vi "Script Constant VI.vi"(7 "Custom Argument Window":refnum<vi>, 8 "error in":errorcluster, 11 "VI Reference":refnum<vi>) -> (0 "error out":errorcluster, 3 "VI reference":refnum<vi>)   [LabVIEW 2019, in "Panther Dashboard.lvlib"]
uses:
  Panther Dashboard.lvlib
  <vilib>/Utility/traverseref.llb/TRef TravTarget.ctl
  <vilib>/Utility/miscctls.llb/LVPositionTypeDef.ctl
  <vilib>/Utility/traverseref.llb/VI Scripting - Traverse.lvlib
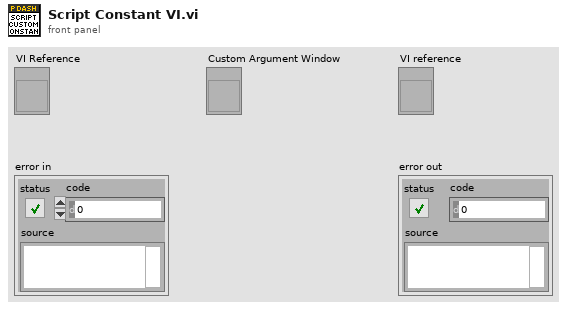
[diagram p1: front panel]
types:
  T1 = typedef "TRef TravTarget.ctl" = enum16{"FP", "BD", "Other"}
  T2 = typedef "LVPositionTypeDef.ctl" = cluster{"Left":i32, "Top":i32}
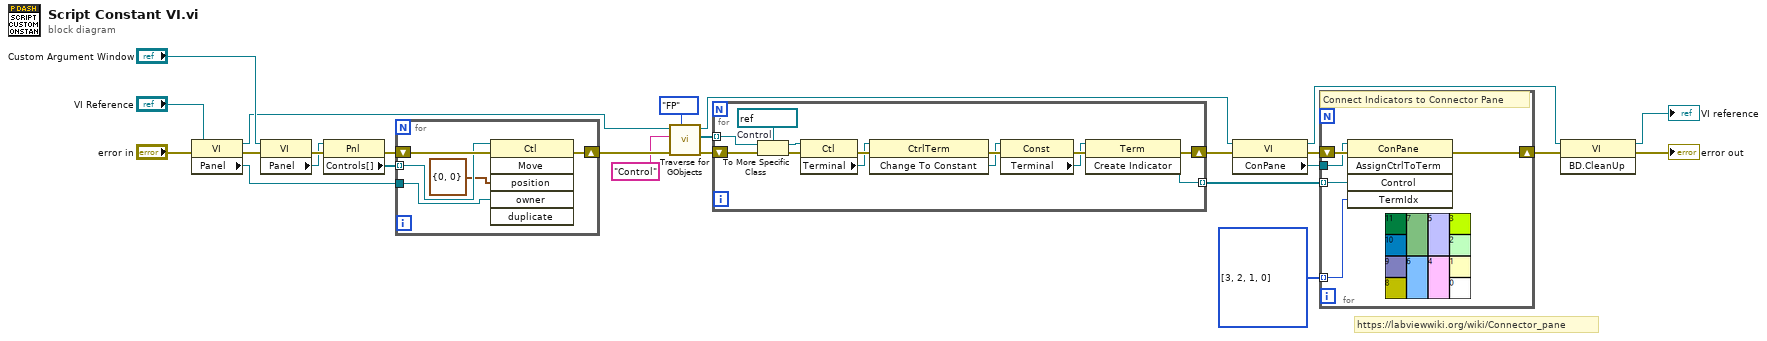
[diagram p0: block diagram]
diagram:
  # "https://labviewwiki.org/wiki/Connector_pane"
  n1 = property class="VI"(reference="VI Reference", error in="error in") -> (reference out=w9:refnum<vi>, error out=w22:errorcluster, "Panel"=w12:refnum<vi>)
  n2 = property class="VI"(reference="Custom Argument Window", error in=w22) -> (error out=w24:errorcluster, "Panel"=w14:refnum<vi>)  [unwired: 1 out]
  n3 = property class="Pnl"(reference=w14, error in=w24) -> (error out=w23:errorcluster, "Controls[]"=w13:refnum<vi>[])  [unwired: 1 out]
  n4 = for {
    tunnel: w13 -> [w28] mode=indexing
    shift-right: [w29] -> w19
    shift-left: w23 -> [w30]
    tunnel: w12 -> [w27]
    n5 = invoke class="Ctl" method="Move"(reference=w28, error in=w30, "position"=T2 {"Left"=0, "Top"=0}, "owner"=w27) -> (error out=w29:errorcluster)  [unwired: 2 in, 5 out]
  }
  n6 = call <vilib>:"Traverse for GObjects.vi"("Traverse Target"=TRef_TravTarget."FP", "error in (no error)"=w19, "Class Name"="Control", "VI Refnum"=w9) -> ("error out"=w17:errorcluster, "References"=w6:refnum<vi>[], "dup VI Refnum"=w8:refnum<vi>)  [unwired: 4 in, 1 out]
  n7 = for {
    tunnel: w6 -> [w33] mode=indexing
    shift-right: [w40] -> w18
    shift-left: w17 -> [w43]
    tunnel: [w36] -> w4 mode=indexing
    w31 = refnum<vi> refnum  # Control
    n8 = To More Specific Class(target class=w31, reference=w33, error in=w43) -> (specific class reference=w32:refnum<vi>, error out=w38:errorcluster)
    n9 = property class="Ctl"(reference=w32, error in=w38) -> (error out=w42:errorcluster, "Terminal"=w37:refnum<vi>)  [unwired: 1 out]
    n10 = invoke class="CtrlTerm" method="Change To Constant"(reference=w37, error in=w42) -> (error out=w41:errorcluster, "Change To Constant"=w35:refnum<vi>)  [unwired: 1 in, 1 out]
    n11 = property class="Const"(reference=w35, error in=w41) -> (error out=w39:errorcluster, "Terminal"=w34:refnum<vi>)  [unwired: 1 out]
    n12 = invoke class="Term" method="Create Indicator"(reference=w34, error in=w39) -> (error out=w40:errorcluster, "Create Indicator"=w36:refnum<vi>)  [unwired: 1 in, 1 out]
  }
  n13 = property class="VI"(reference=w8, error in=w18) -> (reference out=w3:refnum<vi>, error out=w21:errorcluster, "ConPane"=w11:refnum<vi>)
  n14 = for {
    tunnel: w11 -> [w46]
    shift-right: [w47] -> w20
    shift-left: w21 -> [w48]
    tunnel: i32[] [3, 2, 1, 0] -> [w45] mode=indexing
    tunnel: w4 -> [w44] mode=indexing
    # "Connect Indicators to Connector Pane"
    n15 = invoke class="ConPane" method="AssignCtrlToTerm"(reference=w46, error in=w48, "Control"=w44, "TermIdx"=w45) -> (error out=w47:errorcluster)  [unwired: 1 in, 4 out]
  }
  n16 = invoke class="VI" method="BD.CleanUp"(reference=w3, error in=w20) -> (reference out=→"VI reference":refnum<vi>, error out=→"error out":errorcluster)  [unwired: 1 in, 1 out]
